vi "alert.vi"(2 "error in":errorcluster, 3 "device ID":u32 format="%.0x", 4 "Turn on":bool) -> (0 "error out":errorcluster)   [LabVIEW 2017]
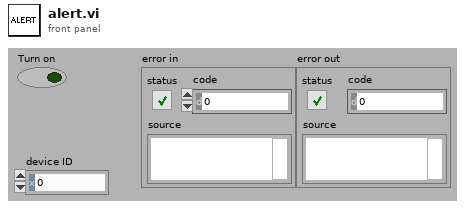
[diagram p1: front panel]
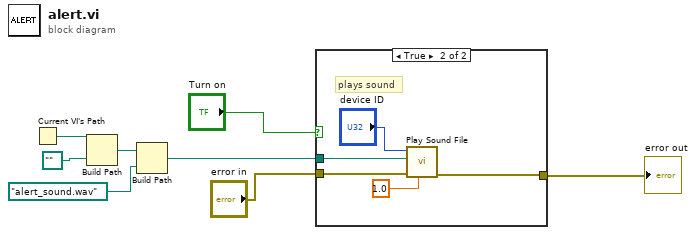
[diagram p0: block diagram]
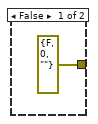
[diagram p2: hidden frame]
diagram:
  n1 = Current VI's Path() -> (path=w5:path)
  n2 = Build Path(base path=w5, name or relative path=path "..") -> (appended path=w3:path)
  n3 = Build Path(base path=w3, name or relative path=path "alert_sound.wav") -> (appended path=w1:path)
  n4 = case shown="True" "Turn on" {
    tunnel: w1 -> [_ w13]
    tunnel: "error in" -> [_ w12]
    tunnel: [errorcluster {"status"=FALSE, "code"=0, "source"=""} ("error out") w10] -> w6
    frame False {
    }
    frame True {
      # "plays sound"
      n5 = call <vilib>:"Play Sound File.vi"("timeout (sec)"=1.0, "error in (no error)"=w12, "path"=w13, "device ID"="device ID") -> ("error out"=w10:errorcluster)  [unwired: 6 in, 1 out]
    }
  }
  "error out" <- w6
